vi "_072.vi"() -> ()   [LabVIEW 2024]
panel:
  out "Duration":u32
  # "Fundamentals :"
  # "~>After running this VI, approximately what is the value displayed in the duration indicator?"
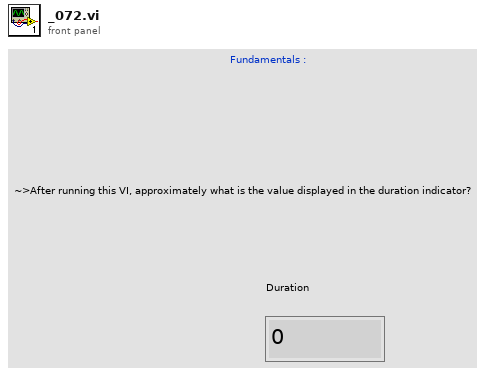
[diagram p1: front panel]
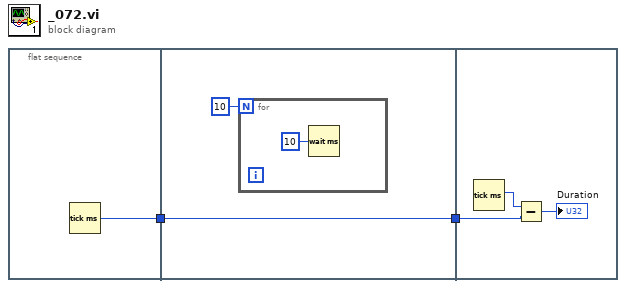
[diagram p0: block diagram]
diagram:
  n1 = flat-sequence {
    tunnel: [w3] -> w1
    tunnel: [w5] -> w2
    tunnel: w1 -> [w5]
    tunnel: w2 -> [w8]
    frame #0 {
      n2 = Tick Count (ms)() -> (millisecond timer value=w3:u32)
    }
    frame #1 {
      n3 = for {
        N: 10 -> [_]
        n4 = Wait (ms)(milliseconds to wait=u32 10) -> ()  [unwired: 1 out]
      }
    }
    frame #2 {
      n5 = Tick Count (ms)() -> (millisecond timer value=w9:u32)
      n6 = Subtract(x=w9, y=w8) -> (x-y=→"Duration":u32)
    }
  }
